vi "GetBDClassCluster.vi"(8 "error in (no error)":errorcluster, 10 "BaseDev Data":T1={"Nom de ressource VISA"="", "DeviceCtrl"=[], "DataNames"=[], "ScanParamOut"=0.0, "HeaderString"="", "Functions"=[], "ScanFuncInd"=0, "Function"="", "StartStatPanel"=FALSE, "PanelVIRef"=refnum, "SubPanelRef"=refnum, "SubPanelCtrl"=[], "LoadedPanelIndex"=-1, "InstrumentName"="", "AvailFuncPan"=["ClassPanel"], "ScanTable"=[], "ScanPanelRef"=refnum, "ScanPanelPath"=path "", "Beforewait(ms)"=0, "Afterwait(ms)"=0, "SynchToClk(ms)"=-1, "FuncPanelIndex"=-1, "ClassQueue"=refnum, "ClassEvent"=refnum, "InstrParam"=[], "DatDisplayNm"=[], "ShowInstrNm"=[], "ShowParSuffix"=[], "ShowScanSuffix"=[], "ShowParValue"=[], "ParSuffix"=[], "ScanSuffix"=[], "Delta Time(ms)"=0, "BaseDataPath"=path "", "SubDatDisplayNm"=[], "SubScanTable(y)"=[], "SubVarParNm X"=[], "SubVarParNm Y"=[], "DataBindCtrl"=[], "DataCtrl"=[], "ReuseVarPar"=FALSE, "LastScanPos"=[], "BackForth"=FALSE, "ArrayDatNm"=[], "ArrayDisplNm"=[]}, 11 "BaseDevice.lvclass":refnum<class "BaseDevice.lvclass">) -> (0 "error out":errorcluster, 3 "BaseDevice.lvclass Out":refnum<class "BaseDevice.lvclass">)   [LabVIEW 2019, in "BaseDevice.lvclass"]
uses:
  BaseDevice.lvclass
  BDClassCluster.ctl
  BaseDevice.lvclass/BaseDevice.ctl
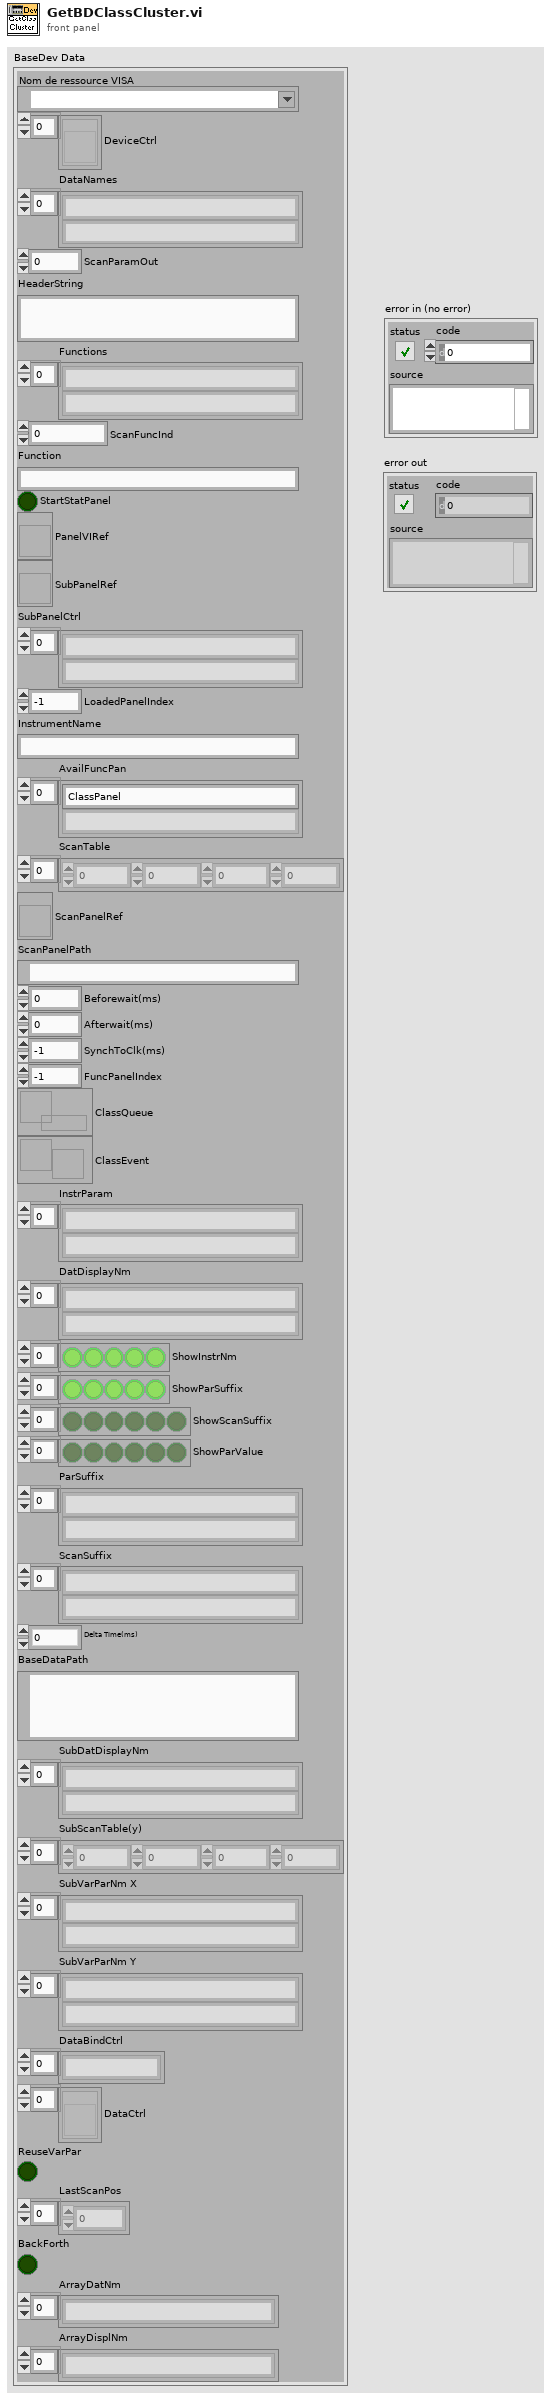
[diagram p1: front panel]
types:
  T1 = typedef "BDClassCluster.ctl" = cluster{"Nom de ressource VISA":refnum<visa-resource-name>, "DeviceCtrl":refnum<vi>[], "DataNames":string[], "ScanParamOut":dbl, "HeaderString":string, "Functions":string[], "ScanFuncInd":i32, "Function":string, "StartStatPanel":bool, "PanelVIRef":refnum<vi>, "SubPanelRef":refnum<vi>, "SubPanelCtrl":string[], "LoadedPanelIndex":i32, "InstrumentName":string, "AvailFuncPan":string[], "ScanTable":dbl[], "ScanPanelRef":refnum<vi>, "ScanPanelPath":path, "Beforewait(ms)":u32, "Afterwait(ms)":u32, "SynchToClk(ms)":i32, "FuncPanelIndex":i32, "ClassQueue":refnum<queue>, "ClassEvent":refnum<user-event>, "InstrParam":string[], "DatDisplayNm":string[], "ShowInstrNm":bool[], "ShowParSuffix":bool[], "ShowScanSuffix":bool[], "ShowParValue":bool[], "ParSuffix":string[], "ScanSuffix":string[], "Delta Time(ms)":u32, "BaseDataPath":path, "SubDatDisplayNm":string[], "SubScanTable(y)":dbl[], "SubVarParNm X":string[], "SubVarParNm Y":string[], "DataBindCtrl":string[], "DataCtrl":refnum<vi>[], "ReuseVarPar":bool, "LastScanPos":dbl[], "BackForth":bool, "ArrayDatNm":string[], "ArrayDisplNm":string[]}
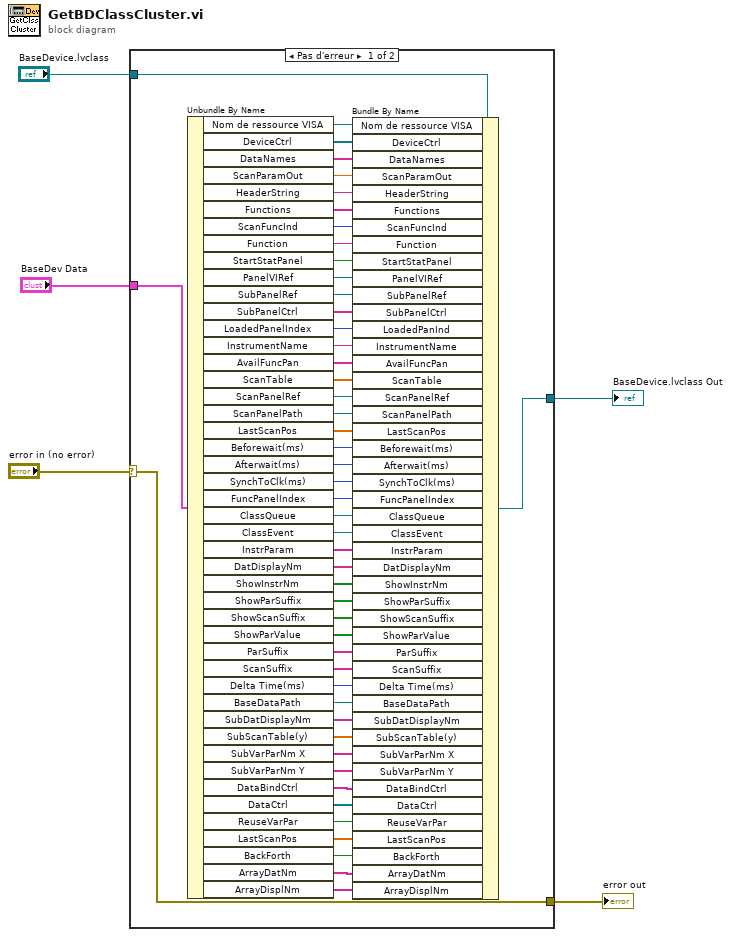
[diagram p0: block diagram]
diagram:
  n1 = case shown="Pas d'erreur" "error in (no error)" {
    selector: "error in (no error)" -> [w55 w56]
    tunnel: "BaseDevice.lvclass" -> [w19 w57]
    tunnel: [w55 w56] -> w3
    tunnel: [w20 w57] -> w2
    tunnel: "BaseDev Data" -> [w21 _]
    frame No Error {
      n2 = Unbundle By Name(w21) -> ("Nom de ressource VISA"=w54:refnum<visa-resource-name>, "DeviceCtrl"=w53:refnum<vi>[], "DataNames"=w52:string[], "ScanParamOut"=w51:dbl, "HeaderString"=w50:string, "Functions"=w49:string[], "ScanFuncInd"=w48:i32, "Function"=w47:string, "StartStatPanel"=w46:bool, "PanelVIRef"=w45:refnum<vi>, "SubPanelRef"=w44:refnum<vi>, "SubPanelCtrl"=w43:string[], "LoadedPanelIndex"=w42:i32, "InstrumentName"=w41:string, "AvailFuncPan"=w40:string[], "ScanTable"=w39:dbl[], "ScanPanelRef"=w22:refnum<vi>, "ScanPanelPath"=w23:path, "LastScanPos"=w24:dbl[], "Beforewait(ms)"=w25:u32, "Afterwait(ms)"=w26:u32, "SynchToClk(ms)"=w27:i32, "FuncPanelIndex"=w28:i32, "ClassQueue"=w29:refnum<queue>, "ClassEvent"=w30:refnum<user-event>, "InstrParam"=w31:string[], "DatDisplayNm"=w32:string[], "ShowInstrNm"=w33:bool[], "ShowParSuffix"=w34:bool[], "ShowScanSuffix"=w35:bool[], "ShowParValue"=w36:bool[], "ParSuffix"=w37:string[], "ScanSuffix"=w38:string[], "Delta Time(ms)"=w18:u32, "BaseDataPath"=w17:path, "SubDatDisplayNm"=w16:string[], "SubScanTable(y)"=w15:dbl[], "SubVarParNm X"=w14:string[], "SubVarParNm Y"=w13:string[], "DataBindCtrl"=w12:string[], "DataCtrl"=w11:refnum<vi>[], "ReuseVarPar"=w10:bool, "LastScanPos"=w9:dbl[], "BackForth"=w8:bool, "ArrayDatNm"=w7:string[], "ArrayDisplNm"=w6:string[])
      n3 = Bundle By Name(cluster=w19, "Nom de ressource VISA"=w54, "DeviceCtrl"=w53, "DataNames"=w52, "ScanParamOut"=w51, "HeaderString"=w50, "Functions"=w49, "ScanFuncInd"=w48, "Function"=w47, "StartStatPanel"=w46, "PanelVIRef"=w45, "SubPanelRef"=w44, "SubPanelCtrl"=w43, "LoadedPanInd"=w42, "InstrumentName"=w41, "AvailFuncPan"=w40, "ScanTable"=w39, "ScanPanelRef"=w22, "ScanPanelPath"=w23, "LastScanPos"=w24, "Beforewait(ms)"=w25, "Afterwait(ms)"=w26, "SynchToClk(ms)"=w27, "FuncPanelIndex"=w28, "ClassQueue"=w29, "ClassEvent"=w30, "InstrParam"=w31, "DatDisplayNm"=w32, "ShowInstrNm"=w33, "ShowParSuffix"=w34, "ShowScanSuffix"=w35, "ShowParValue"=w36, "ParSuffix"=w37, "ScanSuffix"=w38, "Delta Time(ms)"=w18, "BaseDataPath"=w17, "SubDatDisplayNm"=w16, "SubScanTable(y)"=w15, "SubVarParNm X"=w14, "SubVarParNm Y"=w13, "DataBindCtrl"=w12, "DataCtrl"=w11, "ReuseVarPar"=w10, "LastScanPos"=w9, "BackForth"=w8, "ArrayDatNm"=w7, "ArrayDisplNm"=w6) -> (w20:refnum<class "BaseDevice.lvclass">)
    }
    frame Error {
    }
  }
  "BaseDevice.lvclass Out" <- w2
  "error out" <- w3
